vi "Write elements to FIFO and Process on sha.vi"() -> ()   [LabVIEW 2014]
uses:
  <vilib>/rvi/Emulation/niFpgaGetClockAttributes.vi
  <vilib>/rvi/Emulation/niFpgaSctlEmulationGetInTimedLoop.vi
  <vilib>/rvi/Emulation/niFpgaEmulationReportErrorSimple.vi
  <vilib>/rvi/Emulation/niFpgaCriticalErrorInLSC.vi
panel:
  out "FIFO Output":u8[](array[numeric])
  out "Digest":u8[](array[numeric])
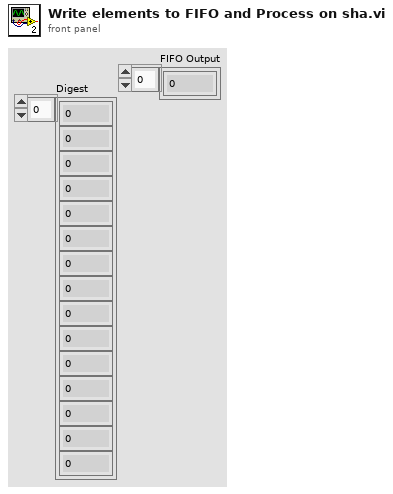
[diagram p1: front panel]
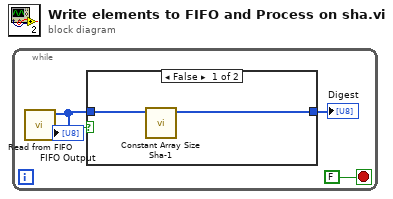
[diagram p0: block diagram]
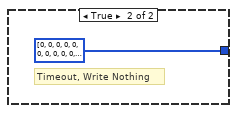
[diagram p2: hidden frame]
diagram:
  n1 = while {
    stop <- FALSE stop-if-true
    n2 = call "Read from FIFO.vi"() -> ("Time Out?"=w3:bool, "Array"=w4:u8[])  [unwired: 10 in]
    "FIFO Output" <- w4
    n3 = case shown="False" w3 {
      tunnel: w4 -> [w6 _]
      tunnel: [w5 u8[] [0, 0, 0, 0, 0, 0, 0, 0, 0, 0, 0, 0, 0, 0, 0, 0, 0, 0, 0, 0] ("Digest")] -> w2
      frame False {
        n4 = call "Constant Array Size Sha-1.vi"("Message In as Byte Array"=w6) -> ("Digest"=w5:u8[])  [unwired: 10 in]
      }
      frame True {
        # "Timeout, Write Nothing"
      }
    }
    "Digest" <- w2
  }
